vi "Close.vi"(8 "error in (no error)":errorcluster, 11 "Event_Syslog in":refnum<class "Event_Syslog.lvclass">) -> (0 "error out":errorcluster, 3 "Event_Syslog out":refnum<class "Event_Syslog.lvclass">)   [LabVIEW 2021, in "Event_Syslog.lvclass"]
uses:
  Event_Syslog.lvclass
  Event_Syslog.lvclass/Event_Syslog.ctl
  abs_EventLog/abs_EventLog.lvclass
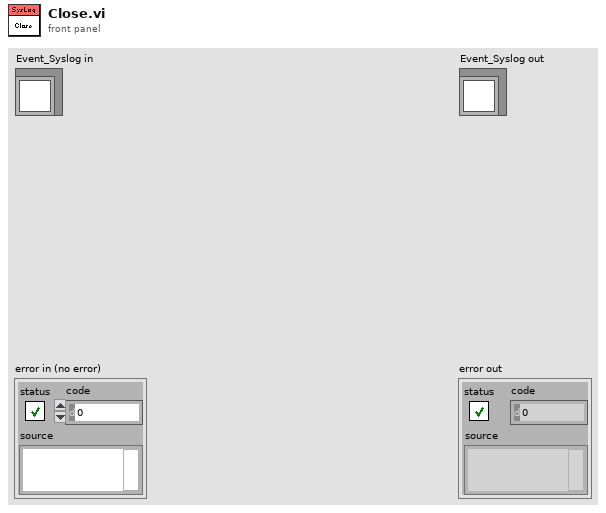
[diagram p1: front panel]
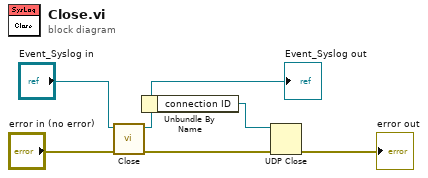
[diagram p0: block diagram]
diagram:
  n1 = call-parent "Close.vi"("error in (no error)"="error in (no error)", "abs_EventLog in"="Event_Syslog in") -> ("error out"=w3:errorcluster, "abs_EventLog out"=w4:refnum<class "Event_Syslog.lvclass">)  [unwired: 8 in]
  "Event_Syslog out" <- w4
  n2 = Unbundle By Name(w4) -> ("connection ID"=w1:refnum<k16>)
  n3 = UDP Close(connection ID=w1, 8:w3) -> (error out=→"error out":errorcluster)  [unwired: 1 out]
